vi "UI - Method Details.vi"(5 "Term (Methods)":string="Methods", 7 "Msg Chain":string, 8 "error in (no error)":errorcluster {"code" format="Error %.0f"}, 10 "UI Docs":refnum<class "GUI Documentation.lvclass">[](array[class]), 11 "VIDoc Printer - Confluence In":refnum<class "VIDoc Printer - Confluence.lvclass">) -> (0 "error out":errorcluster {"code" format="Error %.0f"}, 3 "VIDoc Printer - Confluence Out":refnum<class "VIDoc Printer - Confluence.lvclass">)   [LabVIEW 2023, in "VIDoc Printer - Confluence.lvlib" / "VIDoc Printer - Confluence.lvclass"]
uses:
  VIDoc Printer - Confluence.lvclass
  VIDoc Printer - Confluence.lvclass/VIDoc Printer - Confluence.ctl
  Confluence Formatting/Confluence Formatting.lvlib
  Confluence Formatting/Types/Format Combo Box.ctl
  Parsing/GUI Documentation/GUI Documentation.lvclass
  Types/VI Method Types.ctl
  Printer/VIDoc Printer.lvclass
  C:/projects/DMC/Tooling/Git-Action-Service/Source/Documentation Generation/Printers/Printer/VIDoc Printer.lvclass
  C:/projects/DMC/Tooling/Git-Action-Service/Source/Documentation Generation/Printers/Confluence Printer/VIDoc Printer - Confluence.lvclass
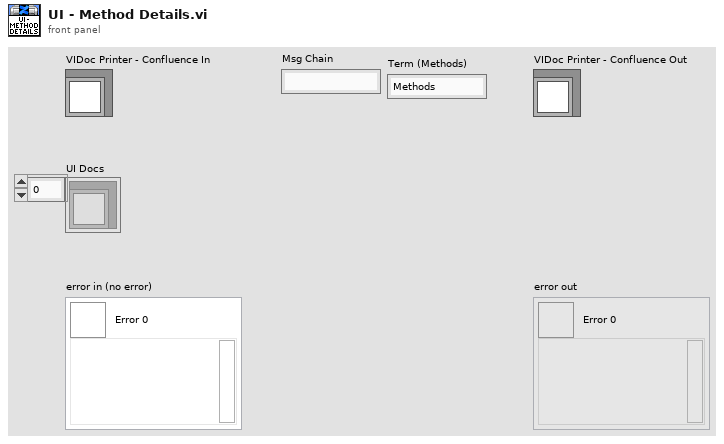
[diagram p1: front panel]
types:
  T1 = typedef "VIDoc Printer - Confluence.lvlib/VIDoc Printer - Confluence.lvclass/VI Method Types.ctl" = enum16{"Library", "Class", "Interface", "LLB", "UI", "List"}
  T2 = typedef "Confluence Formatting.lvlib/Format Combo Box.ctl" = string
  T3 = typedef "VIDoc Printer.lvlib/Printer Settings.lvclass/VI Settings.ctl" = cluster{"Memory":bool, "By Folder":bool, "By Tree":bool, "By List":bool, "Methods":bool, "Method Options":cluster{"Front Panels":bool, "Options":bool, "Controls":bool}, "List Detail Level":T4, "Methods Detail Level":T4, "Controls Detail Level":T4}
  T4 = typedef "VIDoc Printer.lvlib/Printer Settings.lvclass/Detail Level Enum.ctl" = enum16{"None", "Minimal", "Standard", "Full"}
  T5 = typedef "VIDoc Parsing.lvlib/Method Spec Cluster.ctl" = cluster{"VI Type Ext":T6, "Name":string, "Path":path, "Get Conpane Image":T7, "Description":string, "Get Library Access Scope":enum32{"invalid scope", "public", "private", "protected", "community"}, "Dispatch":T8, "ContainsCompiledCode":bool, "Exec.IsReentrant":bool, "Exec.ReentrancyType":enum16{"Share clones between instances", "Preallocate clone for each instance"}, "ExecInlining":bool, "ExecInlineIfPossible":bool, "Auto Err Handling":bool, "CodeComplexity":sgl, "Bookmark Tags":string[], "Control VI Type":enum32{"not a control VI", "control", "typedef", "strict typedef"}, "Controls":T9[], "VI Type":enum32{"invalid VI type", "Standard VI", "Control VI", "Global VI", "Polymorphic VI", "Configuration VI", "SubSystem", "Facade VI", "Method VI", "Statechart Diagram VI"}, "Minimum Size":T11, "Front Panel Window:Title":string, "Front Panel Window:Behavior":enum32{"Invalid", "Default", "Floating", "Floating/Auto-Hide", "Modal"}, "Front Panel Window:Closeable":bool, "Must Override":bool, "Must Use Parent Implementation":bool, "VI Icon":T7, "Front Panel":T7, "History:Revision Number":u32, "Metrics:Total Data Size":u32, "Execution:Allow Debugging":bool, "Execution:Preferred Exec System":enum32{"invalid execution system", "user interface", "standard", "instrument i/o", "data acquisition", "other 1", "other 2", "same as caller"}, "Execution:Priority":enum32{"invalid priority", "background priority", "normal priority", "above normal priority", "high priority", "time critical priority", "subroutine"}, "BM Tag Text":string[], "Block Diagram":T7, "Structure Tree":T12[]}
  T6 = typedef "VIDoc Parsing.lvlib/VI Type Extended Enum.ctl" = enum16{"Unknown", "Class Method", "Class Accessor Get", "Class Accessor Set", "Class Control", "Library Method", "Library Control", "VI", "Control"}
  T7 = typedef "imagedata.ctl" = cluster{"image type":i32, "image depth":i32, "image":u8[], "mask":u8[], "colors":u32[], "Rectangle":cluster{"left":i16, "top":i16, "right":i16, "bottom":i16}}
  T8 = typedef "VIDoc Parsing.lvlib/Class Dispatch Type Enum.ctl" = enum16{"None", "Static", "Dynamic"}
  T9 = typedef "VIDoc Parsing.lvlib/Controls Info Cluster.ctl" = cluster{"Name":string, "Description":string, "Data Type":string, "Tip Strip":string, "UID":i32, "Image Data":T7, "ToggleKeyBind":T10, "Raw Label":string, "Raw Caption":string}
  T10 = typedef "LVKeyTypeDef.ctl" = cluster{"Focus":bool, "Control":bool, "Shift":bool, "Key":string}
  T11 = typedef "LVPointTypeDef.ctl" = cluster{"Horizontal":i16, "Vertical":i16}
  T12 = typedef "VIDoc Parsing.lvlib/Structure Reporter.lvlib/Tree Cluster.ctl" = cluster{"Object Class Name":string, "Labels":string[], "Child Tag":string, "Item Indent":i32, "Child Only?":bool, "Glyph Index":i32}
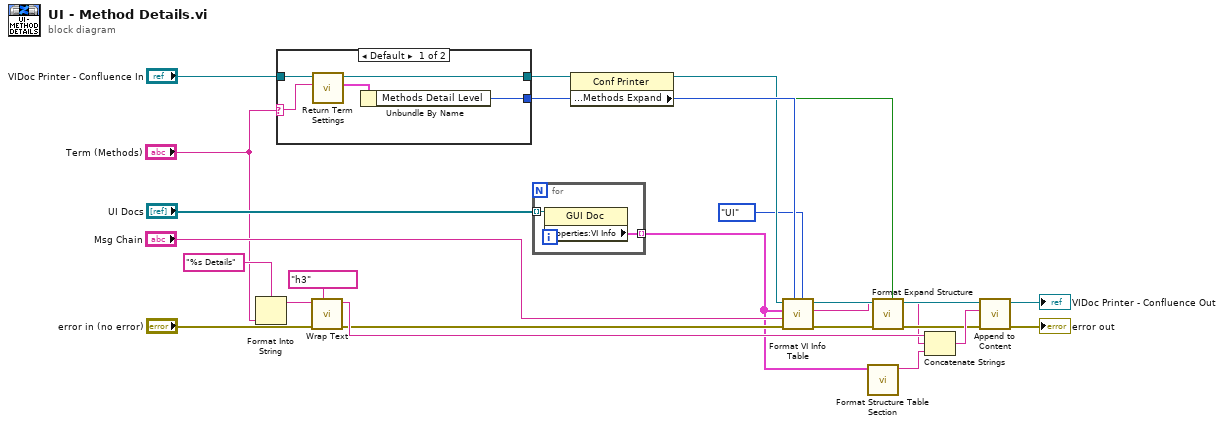
[diagram p0: block diagram]
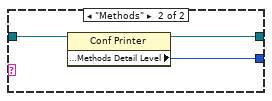
[diagram p2: hidden frame]
diagram:
  n1 = Format Into String(format string="%s Details", "Term (Methods)") -> (resulting string=w20:string)  [unwired: 2 in, 1 out]
  n2 = case shown="Default" "Term (Methods)" {
    selector: "Term (Methods)" -> [w28 _]
    tunnel: "VIDoc Printer - Confluence In" -> [w30 w33]
    tunnel: [w29 w32] -> w15
    tunnel: [w26 w31] -> w10
    frame Default {
      n3 = call "Return Term Settings.vi"("Term"=w28, "Printer in"=w30) -> ("Term Settings"=w27:T3, "Printer out"=w29:refnum<class "VIDoc Printer - Confluence.lvclass">)  [unwired: 7 in, 1 out]
      n4 = Unbundle By Name(w27) -> ("Methods Detail Level"=w26:T4)
    }
    frame "Methods" {
      n5 = property class="Conf Printer"(reference=w33) -> (reference out=w32:refnum<class "VIDoc Printer - Confluence.lvclass">, "Properties:Settings:VI Members:Methods Detail Level"=w31:T4)  [unwired: 1 in, 1 out]
    }
  }
  n6 = call "Wrap Text.vi"("Formatting"=T2 "h3", "Error in"="error in (no error)", "String"=w20) -> ("Error out"=w13:errorcluster, "Wrapped String"=w17:string)  [unwired: 7 in]
  n7 = for {
    tunnel: "UI Docs" -> [w35] mode=indexing
    tunnel: [w34] -> w3 mode=indexing
    n8 = property class="GUI Doc"(reference=w35) -> ("Properties:VI Info"=w34:T5)  [unwired: 1 in, 2 out]
  }
  n9 = property class="Conf Printer"(reference=w15) -> (reference out=w6:refnum<class "VIDoc Printer - Confluence.lvclass">, "Properties:Expand?:VI:Methods Expand"=w5:bool)  [unwired: 1 in, 1 out]
  n10 = call "Format VI Info Table.vi"("Type"=VI_Method_Types."UI", "Methods"=w10, "Error in"=w13, "Msg Chain"="Msg Chain", "VI Info Array"=w3, "VIDoc Printer - Confluence In"=w6) -> ("Error out"=w12:errorcluster, "Table String"=w8:string, "VIDoc Printer - Confluence Out"=w14:refnum<class "VIDoc Printer - Confluence.lvclass">)  [unwired: 3 in]
  n11 = call "Format Structure Table Section.vi"("VI Info Array"=w3) -> ("Section Text"=w2:string)  [unwired: 9 in, 1 out]
  n12 = call "Format Expand Structure.vi"("Enable? (T)"=w5, "Error in"=w12, "Content"=w8) -> ("Error out"=w9:errorcluster, "Expand String"=w7:string)  [unwired: 7 in]
  n13 = Concatenate Strings(w17, w7, w2) -> (w18:string)
  n14 = call "Append to Content.vi"("error in (no error)"=w9, "Content"=w18, "VIDoc Printer - Confluence In"=w14) -> ("error out"=→"error out":errorcluster, "VIDoc Printer - Confluence Out"=→"VIDoc Printer - Confluence Out":refnum<class "VIDoc Printer - Confluence.lvclass">)  [unwired: 7 in]
